vi "gxml_CheckEnumTxt.vi"(7 "EnumNames":string[](array[string]), 8 "error in":errorcluster, 9 "EnumVal":i32, 10 "Item Attributes":string, 11 "Item Name":string) -> (0 "error out":errorcluster)   [LabVIEW 2011, in "Third Party VIs.lvlib" / "GXML.lvlib"]
uses:
  <vilib>/regexp/Match Regular Expression.xnode
  GXML.lvlib
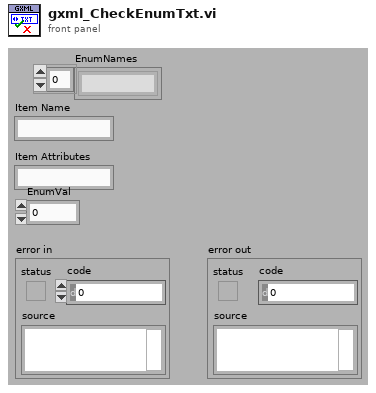
[diagram p1: front panel]
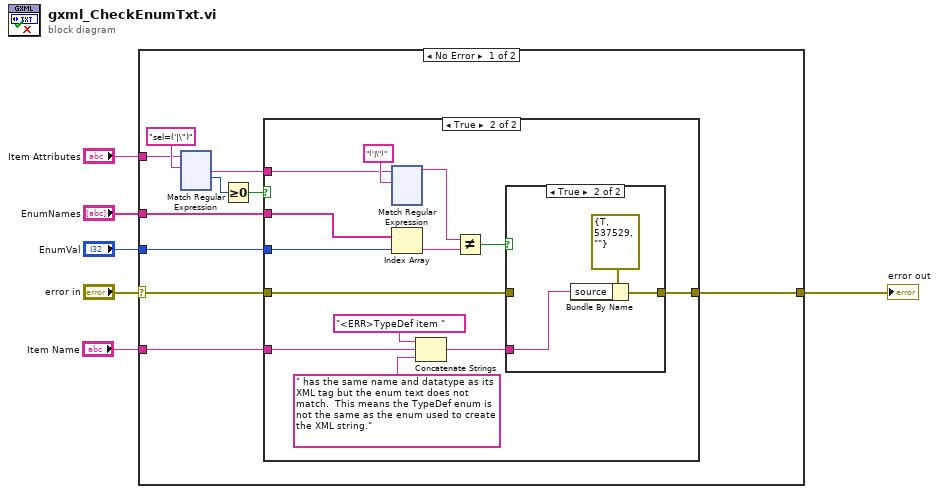
[diagram p0: block diagram]
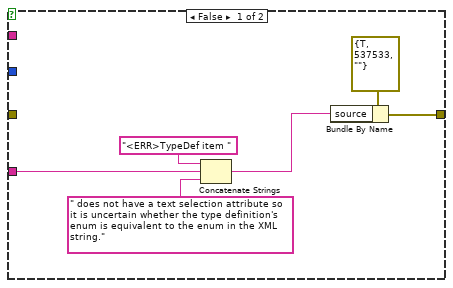
[diagram p2: hidden frame]
diagram:
  n1 = case shown="No Error" "error in" {
    selector: "error in" -> [w11 w262]
    tunnel: [w16 w262] -> w6
    tunnel: "Item Attributes" -> [w8 _]
    tunnel: "EnumVal" -> [w10 _]
    tunnel: "EnumNames" -> [w13 _]
    tunnel: "Item Name" -> [w12 _]
    frame No Error {
      n2 = xnode "Match Regular Expression"("input string"=w8, "regular expression"="sel=('|\")") -> ("after match"=w15:string, "offset past match"=w7:i32)  [unwired: 4 in, 3 out]
      n3 = Greater Or Equal To 0?(x=w7) -> (x >= 0?=w9:bool)
      n4 = case shown="True" w9 {
        tunnel: [w132 w146] -> w16
        tunnel: w15 -> [_ w134]
        tunnel: w13 -> [_ w141]
        tunnel: w12 -> [w128 w139]
        tunnel: w11 -> [_ w136]
        tunnel: w10 -> [_ w135]
        frame False {
          n5 = Concatenate Strings("<ERR>TypeDef item ", w128, " does not have a text selection attribute so it is uncertain whether the type definition's enum is equivalent to the enum in the XML string.") -> (w129:string)
          n6 = Bundle By Name(cluster=errorcluster {"status"=TRUE, "code"=537533, "source"=""} ("error in"), "source"=w129) -> (w132:errorcluster)
        }
        frame True {
          n7 = xnode "Match Regular Expression"("input string"=w134, "regular expression"="('|\")") -> ("before match"=w144:string)  [unwired: 4 in, 4 out]
          n8 = Index Array(array=w141, index=w135) -> (element=w143:string)
          n9 = Concatenate Strings("<ERR>TypeDef item ", w139, " has the same name and datatype as its XML tag but the enum text does not match.  This means the TypeDef enum is not the same as the enum used to create the XML string.") -> (w137:string)
          n10 = Not Equal?(x=w144, y=w143) -> (x != y?=w145:bool)
          n11 = case shown="True" w145 {
            tunnel: w136 -> [w258 _]
            tunnel: [w258 w261] -> w146
            tunnel: w137 -> [_ w259]
            frame False {
            }
            frame True {
              n12 = Bundle By Name(cluster=errorcluster {"status"=TRUE, "code"=537529, "source"=""} ("error in"), "source"=w259) -> (w261:errorcluster)
            }
          }
        }
      }
    }
    frame Error {
    }
  }
  "error out" <- w6
